vi "temp_graph.vi"(11 "file path (dialog if empty) in":path) -> (3 "Curva de temperatura":cluster{"Ramp Pattern":dbl[], u32[]}(graph))   [LabVIEW 2021]
uses:
  <vilib>/Analysis/1siggen.llb/Ramp Pattern by Delta.vi
  <vilib>/Analysis/NI_AALBase.lvlib
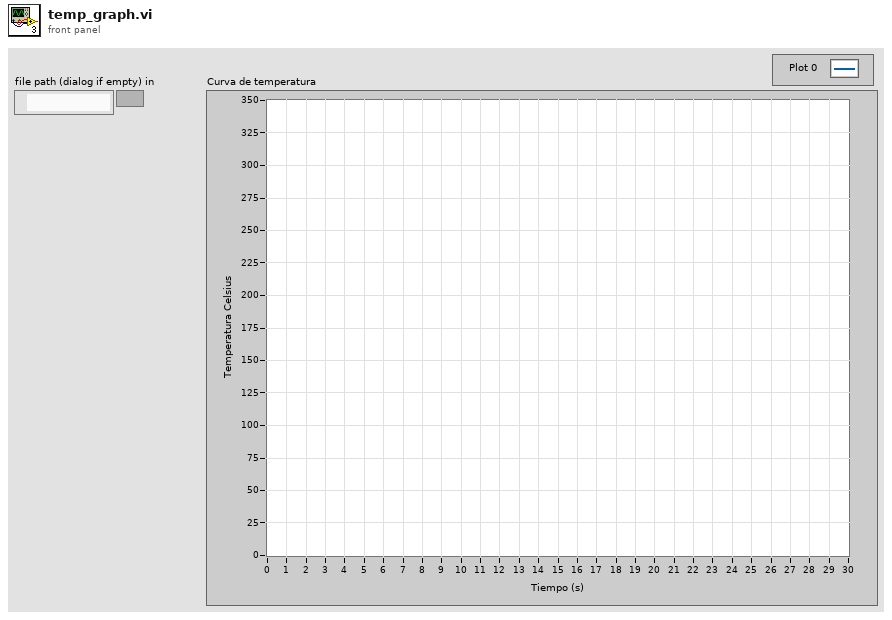
[diagram p1: front panel]
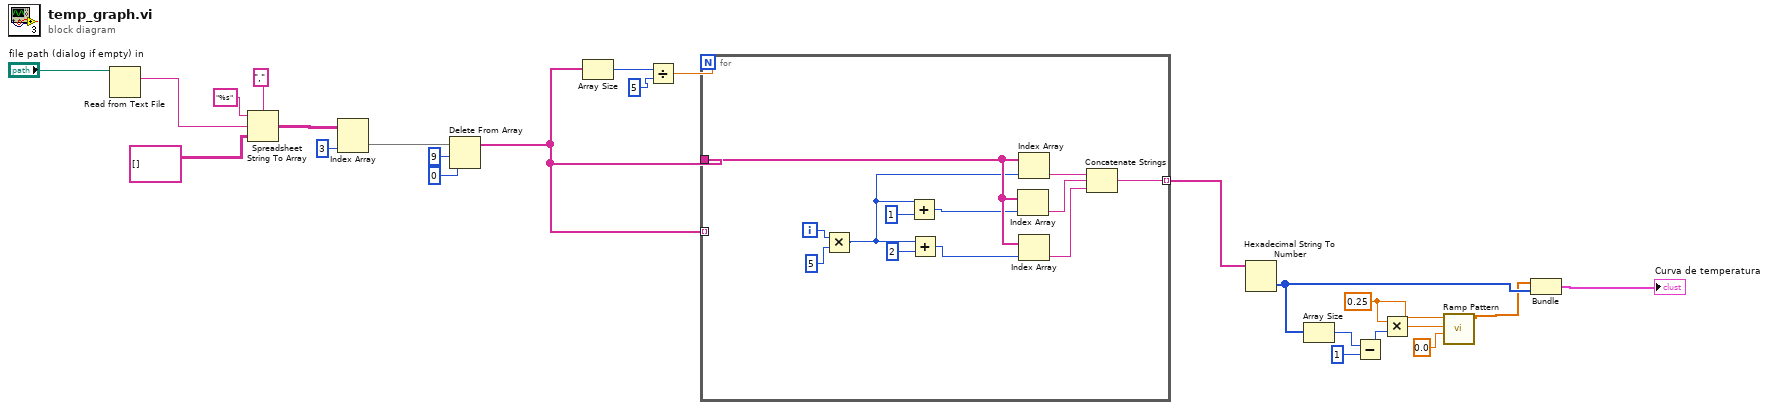
[diagram p0: block diagram]
diagram:
  w5 = 0.25 ("delta")
  n1 = Read from Text File(file (use dialog)="file path (dialog if empty) in") -> (text=w10:string)  [unwired: 3 in, 3 out]
  n2 = Spreadsheet String To Array(delimiter (Tab)=",", format string="%s", spreadsheet string=w10, array type (2D Dbl)=string[][] [] ("Array")) -> (array=w13:string[][])
  n3 = Index Array(array=w13, index (col)=3 ("disabled index (col)")) -> (element=w15:string[])  [unwired: 1 in]
  n4 = Delete From Array(array=w15, length=9, index=0) -> (array with subset deleted=w18:string[])  [unwired: 1 out]
  n5 = Array Size(array=w18) -> (size(s)=w19:i32)
  n6 = Divide(x=w19, y=5) -> (x/y=w21:dbl)
  n7 = for {
    N: w21 -> [_]
    tunnel: w18 -> [_] mode=indexing
    tunnel: w18 -> [w36]
    tunnel: [w32] -> w22 mode=indexing
    i -> [w27]
    n8 = Multiply(x=w27, y=5) -> (x*y=w25:i32)
    n9 = Add(x=w25, y=1) -> (x+y=w29:i32)
    n10 = Add(x=w25, y=2) -> (x+y=w28:i32)
    n11 = Index Array(array=w36, index=w29) -> (element=w34:string)
    n12 = Index Array(array=w36, index=w25) -> (element=w35:string)
    n13 = Index Array(array=w36, index=w28) -> (element=w33:string)
    n14 = Concatenate Strings(w35, w34, w33) -> (w32:string)
  }
  n15 = Hexadecimal String To Number(string=w22) -> (number=w7:u32[])  [unwired: 2 in, 1 out]
  n16 = Array Size(array=w7) -> (size(s)=w3:i32)
  n17 = Subtract(x=w3, y=1) -> (x-y=w1:i32)
  n18 = Multiply(x=w5, y=w1) -> (x*y=w4:dbl)
  n19 = call-poly <vilib>:"Ramp Pattern.vi"("start"=0.0, "end"=w4, "delta"=w5) -> ("Ramp Pattern"=w6:dbl[])  [unwired: 6 in, 2 out]
  n20 = Bundle("Ramp Pattern"=w6, w7) -> (→"Curva de temperatura":cluster{"Ramp Pattern":dbl[], u32[]})  [unwired: 1 in]
